vi "subGetTestStandVersionStringArray.vi"(10 "TestStand Version String":string="[2014, 2016, 2017]") -> (2 "TestStand Version String Array":string[](array[string]))   [LabVIEW 2020, in "veristand-steps-build-tools.lvlib"]
uses:
  veristand-steps-build-tools.lvlib
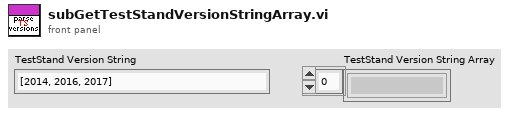
[diagram p1: front panel]
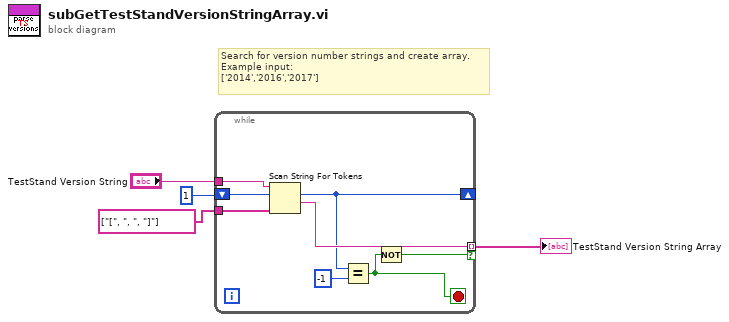
[diagram p0: block diagram]
diagram:
  # "Search for version number strings and create array.\nExample input:\n['2014','2016','2017']"
  n1 = while {
    tunnel: string[] ["[", ", ", "]"] ("delimiters (\\s,\\t,\\r,\\n)") -> [w12]
    shift-right: [w8] -> _
    shift-left: 1 -> [w11]
    tunnel: [w10] -> w3 mode=indexing if=w6
    tunnel: "TestStand Version String" -> [w5]
    stop <- w7 stop-if-true
    n2 = Scan String For Tokens(6:w12, 8:w11, 9:w5) -> (1:w10:string, 2:w8:i32)  [unwired: 3 in, 2 out]
    n3 = Equal?(x=w8, y=-1) -> (x = y?=w7:bool)
    n4 = Not(x=w7) -> (.not. x?=w6:bool)
  }
  "TestStand Version String Array" <- w3
